vi "Logica del negocio.vi"(8 "Module ID":i32=-1, 10 "Seleccion Producto Actual":T1, 11 "Credito":dbl) -> ()   [LabVIEW 2020, in "ControllerUI.lvlib"]
uses:
  ControllerUI.lvlib
  ProductControl/Seleccion Producto Actualizada Argument--cluster.ctl
  <vilib>/PantherLAB/Message Module/Libraries/Message/PantherLAB_lib_Message.lvlib
  MoneyControl/MoneyControl.lvlib
  ProductControl/ProductControl.lvlib
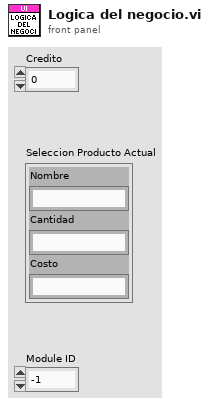
[diagram p1: front panel]
types:
  T1 = typedef "ProductControl.lvlib/Seleccion Producto Actualizada Argument--cluster.ctl" = cluster{"Nombre":string, "Cantidad":string, "Costo":string}
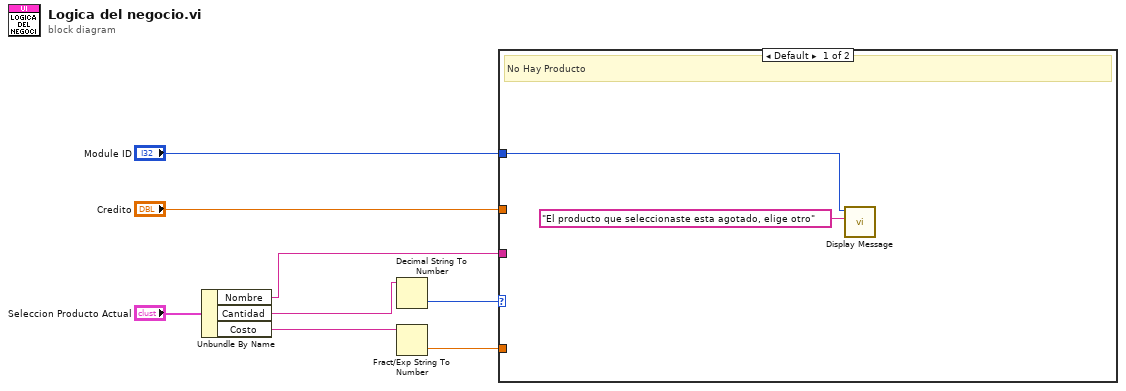
[diagram p0: block diagram]
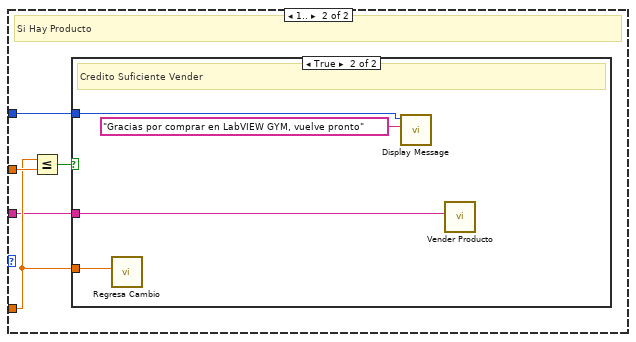
[diagram p2: hidden frame]
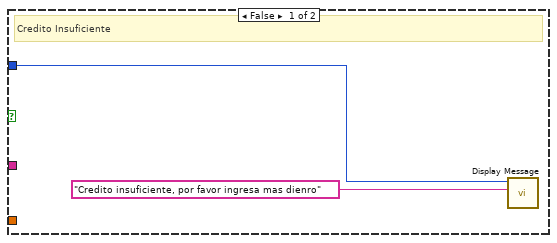
[diagram p3: hidden frame]
diagram:
  n1 = Unbundle By Name("Seleccion Producto Actual") -> ("Nombre"=w1:string, "Cantidad"=w3:string, "Costo"=w2:string)
  n2 = Decimal String To Number(string=w3) -> (number=w8:i32)  [unwired: 2 in, 1 out]
  n3 = Fract/Exp String To Number(string=w2) -> (number=w7:dbl)  [unwired: 3 in, 1 out]
  n4 = case shown="Default" w8 {
    tunnel: w7 -> [_ w12]
    tunnel: "Credito" -> [_ w15]
    tunnel: "Module ID" -> [w9 w13]
    tunnel: w1 -> [_ w11]
    frame Default {
      # "No Hay Producto"
      n5 = call <vilib>:"Display Message.vi"("Message"="El producto que seleccionaste esta agotado, elige otro", "Module ID"=w9) -> ()  [unwired: 9 in, 1 out]
    }
    frame 1.. {
      # "Si Hay Producto"
      n6 = Less Or Equal?(x=w12, y=w15) -> (x <= y?=w14:bool)
      n7 = case shown="True" w14 {
        tunnel: w13 -> [w17 w19]
        tunnel: w12 -> [_ w21]
        tunnel: w11 -> [_ w18]
        frame False {
          # "Credito Insuficiente"
          n8 = call <vilib>:"Display Message.vi"("Message"="Credito insuficiente, por favor ingresa mas dienro", "Module ID"=w17) -> ()  [unwired: 9 in, 1 out]
        }
        frame True {
          # "Credito Suficiente Vender"
          n9 = call "Regresa Cambio.vi"("Costo Producto vendido"=w21) -> ()  [unwired: 10 in, 1 out]
          n10 = call <vilib>:"Display Message.vi"("Message"="Gracias por comprar en LabVIEW GYM, vuelve pronto", "Module ID"=w19) -> ()  [unwired: 9 in, 1 out]
          n11 = call "Vender Producto.vi"("Nombre Producto"=w18) -> ()  [unwired: 10 in, 1 out]
        }
      }
    }
  }
